vi "Ejercicio 3.1.vi"() -> ()   [LabVIEW 2020]
uses:
  <vilib>/numeric/Random Number (Range) DBL.vi
panel:
  out "C° y EMA":cluster{dbl[]}[](graph)
  in  "stop":bool
  out "min value":dbl
  out "max value":dbl
  out "Filtro EMA":dbl[](graph)
  out "?":dbl[][](array[numeric])
  out "Valores aleatoreos de la temperatura C°":dbl[](graph)
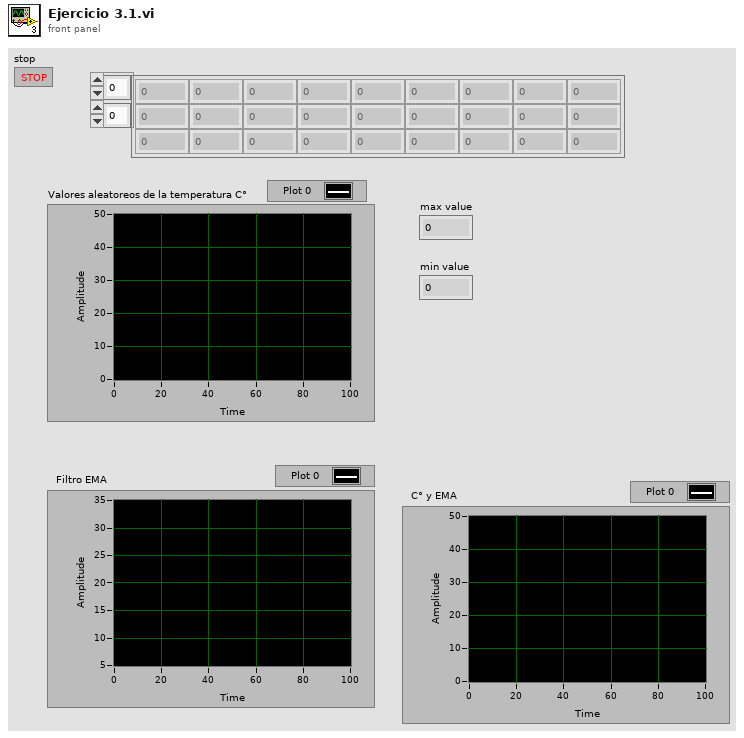
[diagram p1: front panel]
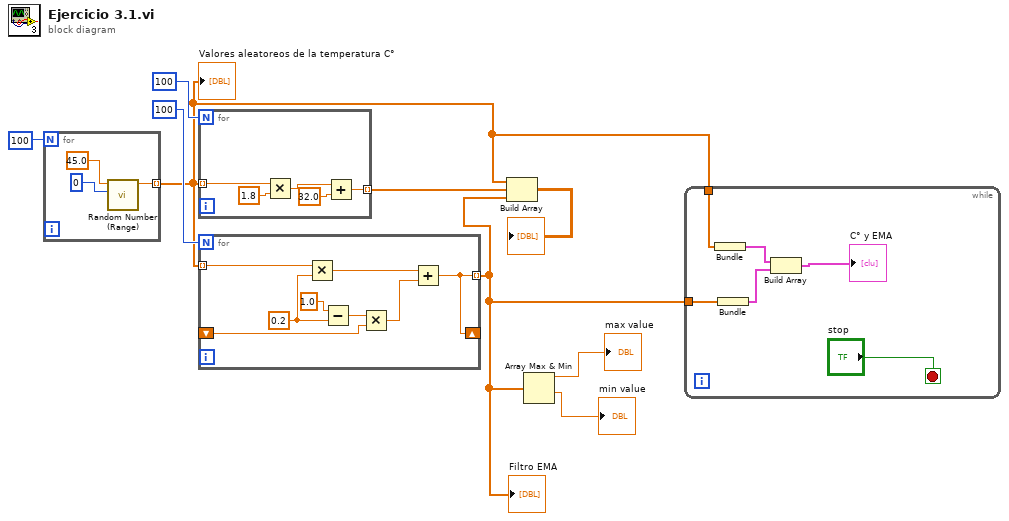
[diagram p0: block diagram]
diagram:
  n1 = for {
    N: 100 -> [_]
    tunnel: [w10] -> w2 mode=indexing
    n2 = call-poly <vilib>:"Random Number (Range).vi"("lower bound (0)"=u64 0, "upper bound (100)"=45.0) -> ("number"=w10:dbl)  [unwired: 9 in]
  }
  "Valores aleatoreos de la temperatura C°" <- w2
  n3 = for {
    N: 100 -> [_]
    tunnel: w2 -> [w17] mode=indexing
    tunnel: [w13] -> w3 mode=indexing
    n4 = Multiply(x=w17, y=1.8) -> (x*y=w15:dbl)
    n5 = Add(x=w15, y=32.0) -> (x+y=w13:dbl)
  }
  n6 = for {
    N: 100 -> [_]
    shift-right: [w19] -> _
    shift-left: _ -> [w20]
    tunnel: [w19] -> w1 mode=indexing
    tunnel: w2 -> [w18] mode=indexing
    w23 = 0.2 ("y")
    n7 = Multiply(x=w18, y=w23) -> (x*y=w25:dbl)
    n8 = Subtract(x=1.0, y=w23) -> (x-y=w22:dbl)
    n9 = Multiply(x=w22, y=w20) -> (x*y=w21:dbl)
    n10 = Add(x=w25, y=w21) -> (x+y=w19:dbl)
  }
  "Filtro EMA" <- w1
  n11 = Build Array(w2, w3, w1) -> (→"?":dbl[][])
  n12 = Array Max & Min(array=w1) -> (max value=→"max value":dbl, min value=→"min value":dbl)  [unwired: 2 out]
  n13 = while {
    tunnel: w2 -> [w30]
    tunnel: w1 -> [w29]
    stop <- "stop" stop-if-true
    n14 = Bundle(w30) -> (w27:cluster{dbl[]})  [unwired: 1 in]
    n15 = Bundle(w29) -> (w28:cluster{dbl[]})  [unwired: 1 in]
    n16 = Build Array(w27, w28) -> (→"C° y EMA":cluster{dbl[]}[])
  }
